vi "Read External Logging Data.vi"(8 "error in (no error)":errorcluster, 10 "Maximum Number of Records":u32, 11 "VISA resource name":refnum<visa-resource-name>) -> (0 "error out":errorcluster, 2 "Records":dbl[](array[numeric]), 3 "VISA resource name out":refnum<visa-resource-name>)   [LabVIEW 2021, in "Agilent N6900 N7900 Series.lvlib"]
doc: "Returns the most recent external datalog records. Data must be read from the buffer periodically to avoid the buffer overflowing. \n\nNote: This VI is not valid in N6900 models."
uses:
  <instrlib>/Agilent N6900 N7900 Series/Agilent N6900 N7900 Series.lvlib
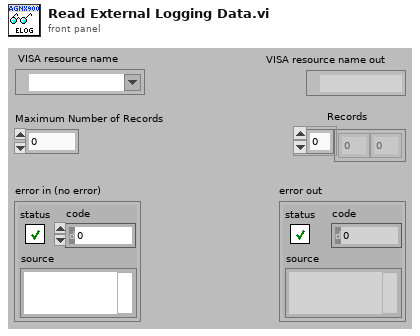
[diagram p1: front panel]
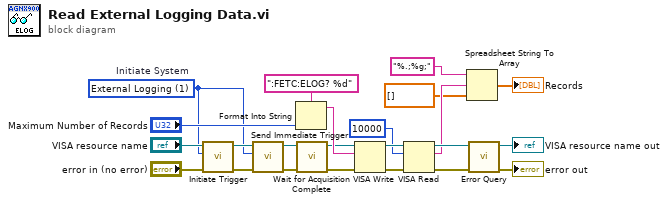
[diagram p0: block diagram]
diagram:
  w1 = u16 1 items=["Acquisition", "External Logging", "Transient"]  # Initiate System
  n1 = call <instrlib>:"Initiate Trigger.vi"("error in (no error)"="error in (no error)", "Initiate System (0: Acquisition)"=w1, "VISA resource name"="VISA resource name") -> ("error out"=w6:errorcluster, "VISA resource name out"=w7:refnum<visa-resource-name>)  [unwired: 7 in]
  n2 = call <instrlib>:"Send Immediate Trigger.vi"("error in (no error)"=w6, "Trigger System (0: Acquisition)"=w1, "VISA resource name"=w7) -> ("error out"=w4:errorcluster, "VISA resource name out"=w5:refnum<visa-resource-name>)  [unwired: 7 in]
  n3 = Format Into String(format string=":FETC:ELOG? %d", "Maximum Number of Records") -> (resulting string=w15:string)  [unwired: 2 in, 1 out]
  n4 = call <instrlib>:"Wait for Acquisition Complete.vi"("error in (no error)"=w4, "VISA resource name"=w5) -> ("error out"=w3:errorcluster, "VISA resource name out"=w2:refnum<visa-resource-name>)  [unwired: 8 in]
  n5 = VISA Write(VISA resource name=w2, write buffer=w15, error in (no error)=w3) -> (VISA resource name out=w19:refnum<visa-resource-name>, error out=w18:errorcluster)  [unwired: 1 out]
  n6 = VISA Read(VISA resource name=w19, byte count=u32 10000, error in (no error)=w18) -> (VISA resource name out=w20:refnum<visa-resource-name>, read buffer=w13:string, error out=w21:errorcluster)  [unwired: 1 out]
  n7 = Spreadsheet String To Array(format string="%.;%g;", spreadsheet string=w13, array type (2D Dbl)=dbl[] []) -> (array=→"Records":dbl[])  [unwired: 1 in]
  n8 = call <instrlib>:"Error Query.vi"("error in (no error)"=w21, "VISA resource name"=w20) -> ("error out"=→"error out":errorcluster, "VISA resource name out"=→"VISA resource name out":refnum<visa-resource-name>)  [unwired: 6 in, 2 out]
